vi "RichToFlatnidaqmx_grpc_ReadCounterScalarF64Response.vi"(5 "OutputClusterType":T1, 11 "InputCluster":T2) -> (3 "OutputCluster":T1)   [LabVIEW 2021, in "NI_DAQmx_client.lvlib"]
uses:
  nidaqmx_grpc_ReadCounterScalarF64Response.ctl
  nidaqmx_grpc_ReadCounterScalarF64Response_Flat.ctl
  NI_DAQmx_client.lvlib
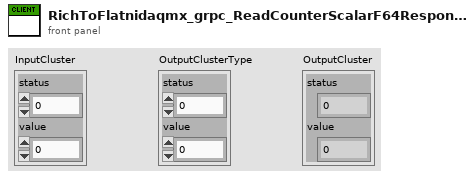
[diagram p1: front panel]
types:
  T1 = typedef "NI_DAQmx_client.lvlib/nidaqmx_grpc_ReadCounterScalarF64Response_Flat.ctl" = cluster{"status":i32, "value":dbl}
  T2 = typedef "NI_DAQmx_client.lvlib/nidaqmx_grpc_ReadCounterScalarF64Response.ctl" = cluster{"status":i32, "value":dbl}
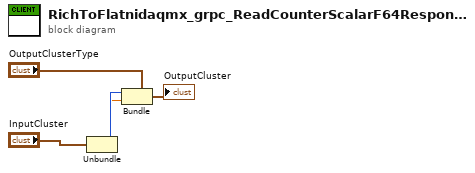
[diagram p0: block diagram]
diagram:
  n1 = Unbundle "Unbundle"("InputCluster") -> ("status"=w2:i32, "value"=w1:dbl)
  n2 = Bundle "Bundle"(cluster="OutputClusterType", "status"=w2, "value"=w1) -> (→"OutputCluster":T1)
